vi "Dereference Bitmap.vi"(5 "Back":u32(colorbox)=16448250, 7 "Front":u32(colorbox), 8 "error in (no error)":errorcluster, 11 "bitmap":T2) -> (0 "error out":errorcluster, 3 "image data":T1)   [LabVIEW 2023, in "Freetype Drawer.lvlib"]
uses:
  Freetype Drawer.lvlib
  FT Bitmap.ctl
  <vilib>/picture/picture.llb/imagedata.ctl
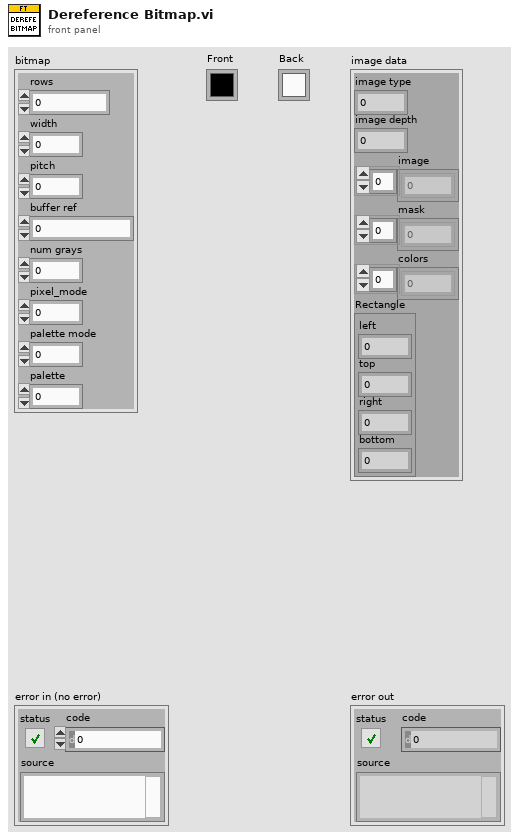
[diagram p1: front panel]
types:
  T1 = typedef "imagedata.ctl" = cluster{"image type":i32, "image depth":i32, "image":u8[], "mask":u8[], "colors":u32[], "Rectangle":cluster{"left":i16, "top":i16, "right":i16, "bottom":i16}}
  T2 = typedef "Freetype Drawer.lvlib/FT Bitmap.ctl" = cluster{"rows":u32, "width":u32, "pitch":i32, "buffer ref":i64, "num grays":i16, "pixel_mode":u8, "palette mode":u8, "palette":i64}
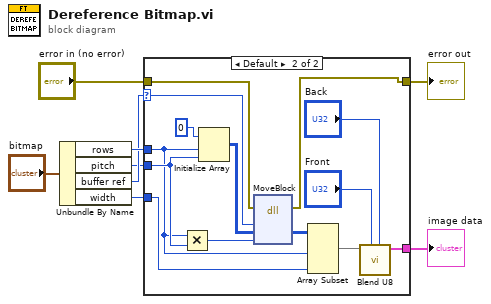
[diagram p0: block diagram]
diagram:
  n1 = Unbundle By Name("bitmap") -> ("rows"=w5:u32, "pitch"=w3:i32, "buffer ref"=w4:i64, "width"=w1:u32)
  n2 = case shown="Default" w4 {
    selector: w4 -> [_ w21]
    tunnel: [w9 w23] -> w8
    tunnel: "error in (no error)" -> [w9 w22]
    tunnel: w5 -> [_ w10]
    tunnel: w3 -> [_ w19]
    tunnel: [_ w16] -> w2
    tunnel: w1 -> [_ w11]
    frame 0 {
    }
    frame Default {
      n3 = Multiply(x=w10, y=w19) -> (x*y=w18:u32)
      n4 = Initialize Array(u8 0 ("Numeric"), w10, w19) -> (w20:u8[][])
      n5 = dll-call lib="LabVIEW" fn="MoveBlock"(error in=w22, "in"=w21, "out"=w20, "size"=w18) -> (error out=w23:errorcluster, "out"=w17:u8[][])  [unwired: 5 in, 1 out]
      n6 = Array Subset(array=w17, length (row)=w10, length (col)=w11) -> (w13:u8[][])  [unwired: 2 in]
      n7 = call "Blend U8.vi"("Back"="Back", "Front"="Front", "U8"=w13) -> ("image data"=w16:T1)  [unwired: 8 in]
    }
  }
  "error out" <- w8
  "image data" <- w2
